vi "WriteReadErrorHandler(SubVI).vi"(8 "error in (no error)":errorcluster, 11 "Parameter Out in":T1) -> (0 "error out":errorcluster, 3 "Parameter Out out":T1)   [LabVIEW 2017, in "LV_Unicorn.lvlib"]
uses:
  LV_Unicorn.lvlib
  Control/unicorn_conn.ctl
  <vilib>/Utility/error.llb/DialogType.ctl
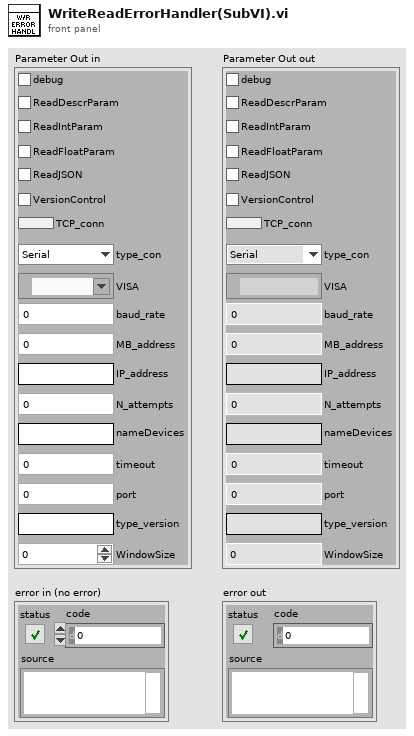
[diagram p1: front panel]
types:
  T1 = typedef "LV_Unicorn.lvlib/unicorn_conn.ctl" = cluster{"ReadIntParam":bool, "ReadDescrParam":bool, "ReadFloatParam":bool, "debug":bool, "ReadJSON":bool, "IP_address":string, "N_attempts":i32, "type_con":enum16{"Serial", "TCP"}, "MB_address":i32, "VISA":refnum<visa-resource-name>, "connection ID":refnum<k5>, "nameDevices":string, "timeout":i32, "port":u16, "type_version":string, "baud_rate":u32, "VersionControl":bool, "TCP_conn":bool, "WindowSize":i32}
  T2 = typedef "DialogType.ctl" = u16
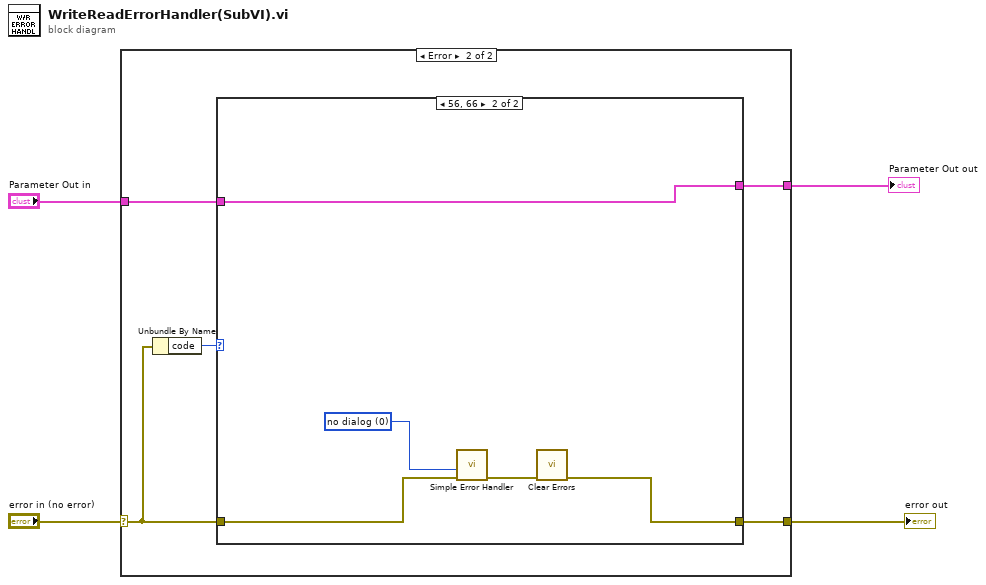
[diagram p0: block diagram]
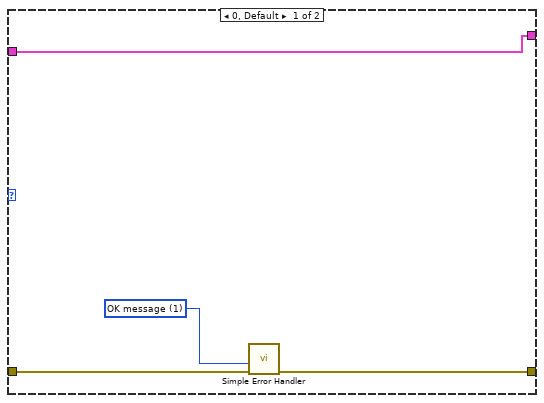
[diagram p3: hidden frame]
diagram:
  n1 = case shown="Error" "error in (no error)" {
    selector: "error in (no error)" -> [w6 w10]
    tunnel: [w6 w9] -> w4
    tunnel: "Parameter Out in" -> [w5 w8]
    tunnel: [w5 w7] -> w3
    frame No Error {
    }
    frame Error {
      n2 = Unbundle By Name(w10) -> ("code"=w11:i32)
      n3 = case shown="56, 66" w11 {
        tunnel: w10 -> [w14 w20]
        tunnel: [w13 w16] -> w9
        tunnel: w8 -> [w15 w18]
        tunnel: [w15 w18] -> w7
        frame 0, Default {
          w12 = T2 1 items=["no dialog", "OK message", "continue or stop message", "OK message + warnings", "continue/stop + warnings"] ("type of dialog (OK msg:1)")
          n4 = call <vilib>:"Simple Error Handler.vi"("type of dialog (OK msg:1)"=w12, "error in (no error)"=w14) -> ("error out"=w13:errorcluster)  [unwired: 3 in, 4 out]
        }
        frame 56, 66 {
          w19 = T2 0 items=["no dialog", "OK message", "continue or stop message", "OK message + warnings", "continue/stop + warnings"] ("type of dialog (OK msg:1)")
          n5 = call <vilib>:"Simple Error Handler.vi"("type of dialog (OK msg:1)"=w19, "error in (no error)"=w20) -> ("error out"=w17:errorcluster)  [unwired: 3 in, 4 out]
          n6 = call <vilib>:"Clear Errors.vi"("error in (no error)"=w17) -> ("error out"=w16:errorcluster)  [unwired: 5 in, 1 out]
        }
      }
    }
  }
  "error out" <- w4
  "Parameter Out out" <- w3
